vi "AFM_Driver_Manager.SendRun.vi"(8 "error in (no error)":errorcluster, 11 "AFM_Driver_Manager in":refnum<class "AFM_Driver_Manager.lvclass">) -> (0 "error out":errorcluster, 3 "AFM_Driver_Manager out":refnum<class "AFM_Driver_Manager.lvclass">)   [LabVIEW 2019, in "AFM_Driver_Manager.lvclass"]
uses:
  AFM_Driver_Manager.lvclass
  AFM_Driver_Manager.lvclass/AFM_Driver_Manager.ctl
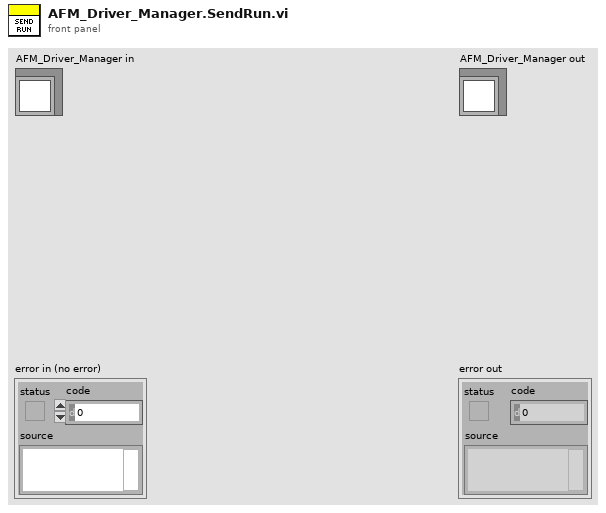
[diagram p1: front panel]
types:
  T1 = typedef "AFM_Driver_Manager.lvclass/AFM_Driver_Manager.PublicMethods.ctl" = cluster{"Stop Event":refnum<user-event>, "Lithography Data":refnum<user-event>, "Run Lithography":refnum<user-event>, "Background Image":refnum<user-event>, "Abort Notifier":refnum<user-event>}
  T2 = cluster{"VI Refnum":refnum<vi>, "Path":path, "Name":string, "Events":T1}
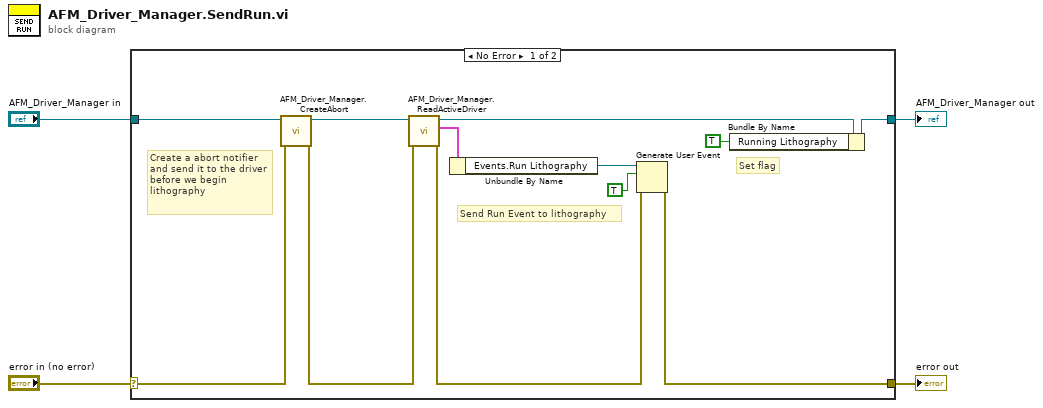
[diagram p0: block diagram]
diagram:
  n1 = case shown="No Error" "error in (no error)" {
    selector: "error in (no error)" -> [w9 w18]
    tunnel: [w12 w18] -> w3
    tunnel: [w6 w17] -> w1
    tunnel: "AFM_Driver_Manager in" -> [w10 w17]
    frame No Error {
      # "Send Run Event to lithography"
      # "Set flag"
      # "Create a abort notifier and send it to the driver before we begin lithography"
      n2 = call "AFM_Driver_Manager.CreateAbort.vi"("error in (no error)"=w9, "AFM_Driver_Manager in"=w10) -> ("error out"=w8:errorcluster, "AFM_Driver_Manager out"=w11:refnum<class "AFM_Driver_Manager.lvclass">)  [unwired: 8 in]
      n3 = call "AFM_Driver_Manager.ReadActiveDriver.vi"("error in (no error)"=w8, "AFM_Driver_Manager in"=w11) -> ("error out"=w13:errorcluster, "Active Driver"=w16:T2, "AFM_Driver_Manager out"=w7:refnum<class "AFM_Driver_Manager.lvclass">)  [unwired: 7 in]
      n4 = Unbundle By Name(w16) -> ("Events.Run Lithography"=w15:refnum<user-event>)
      n5 = Generate User Event(user event=w15, event data cluster=TRUE ("event data"), error in=w13) -> (error out=w12:errorcluster)  [unwired: 1 in, 1 out]
      n6 = Bundle By Name(cluster=w7, "Running Lithography"=TRUE) -> (w6:refnum<class "AFM_Driver_Manager.lvclass">)
    }
    frame Error {
    }
  }
  "error out" <- w3
  "AFM_Driver_Manager out" <- w1
